vi "Element Edit.vi"(10 "Data":T1, 11 "Project":string) -> (2 "Data Out":T1, 3 "OK?":bool)   [LabVIEW 2020]
uses:
  Global/Data Global/SDQ Data Type.ctl
panel:
  in  "Cancle":bool
  in  "OK":bool
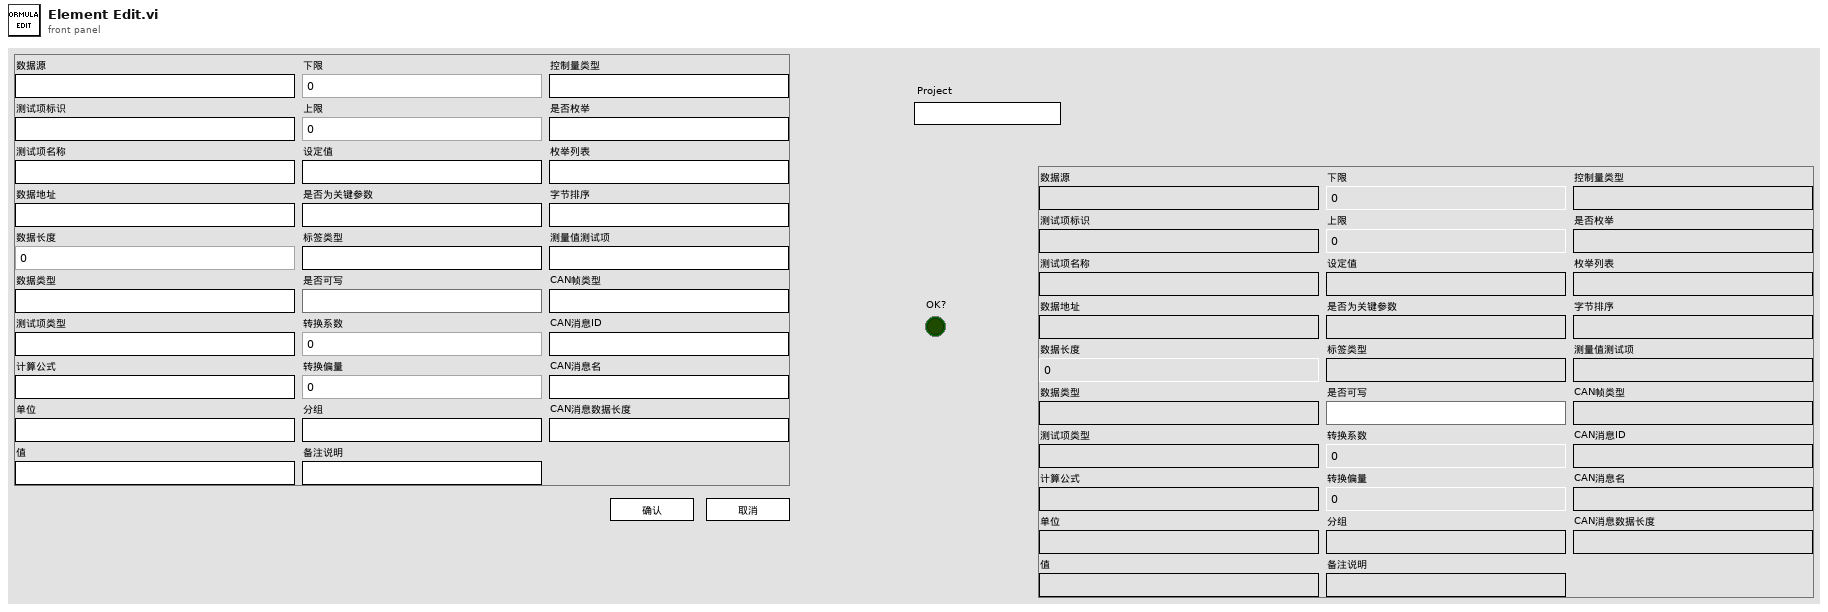
[diagram p1: front panel]
types:
  T1 = typedef "SDQ Data Type.ctl" = cluster{"CAN Length":string, "CAN Name":string, "CAN ID":string, "CAN Type":string, "Test Item":string, "Byte Order":string, "Instruction":string, "Control Type":string, "Group":string, "Offset":dbl, "Coefficient":dbl, "Write Enable":bool, "Lable Type":string, "Key?":string, "Set Value":string, "Upper":dbl, "Lower":dbl, "Unit":string, "Formula":string, "Test Item Type":string, "Length":i32, "Address":string, "Name":string, "Identifier":string, "Data Type":string, "Enumerate?":string, "Enumerate List":string, "Data":string, "Source":string}
  T2 = typedef "eventvkey.ctl" = enum16{"ASCII", "Enter", "Return", "Shift", "Ctrl", "Alt", "Cmd", "Opt", "Caps", "NumLock", "Clear", "Break", "Up", "Down", "Left", "Right", "Insert", "Delete", "Home", "End", "PageUp", "PageDown", "Escape", "Help", "Pause", "ScrollLock", "F1", "F2", "F3", "F4", "F5", "F6", "F7", "F8", "F9", "F10", "F11", "F12", "F13", "F14", "F15", "F16", "F17", "F18", "F19", "F20", "F21", "F22", "F23", "F24", "Play", "VolumeUp", "VolumeDown", "Mute", "Two Byte Char"}
  T3 = cluster{"Project":string, "Element":T1, "OK?":bool}
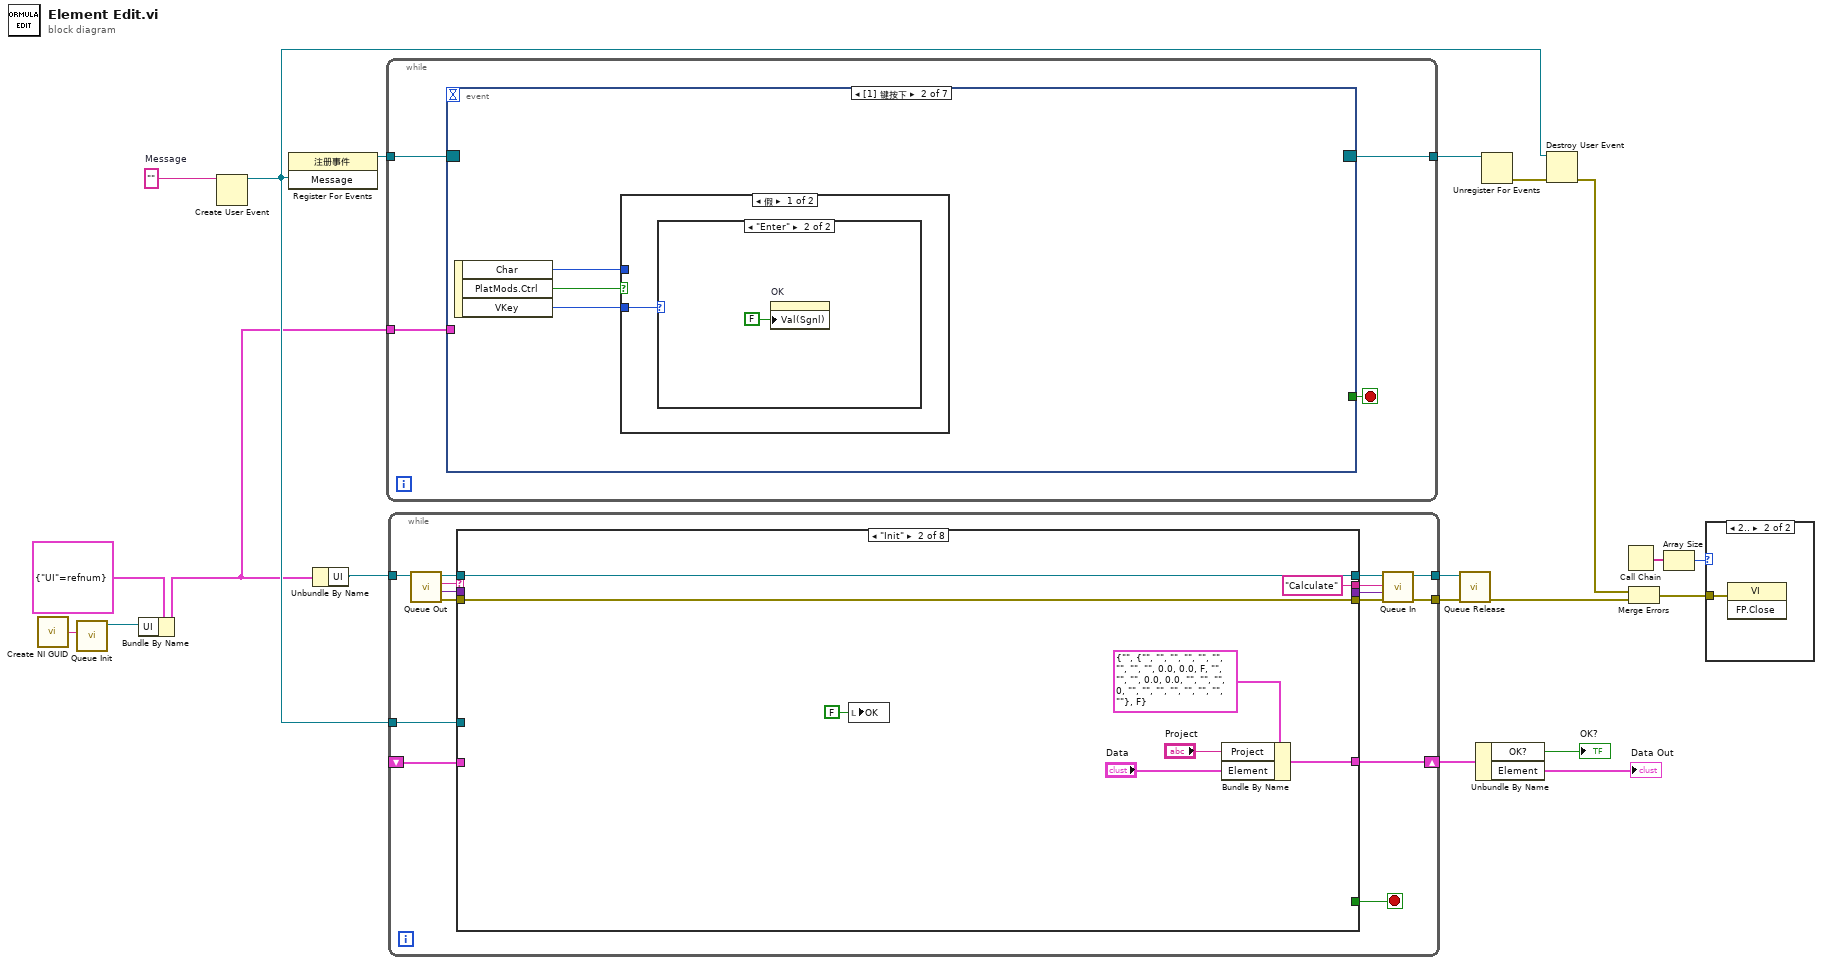
[diagram p0: block diagram]
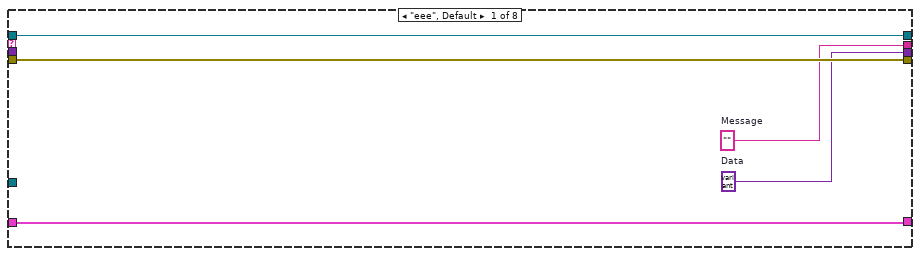
[diagram p3: hidden frame]
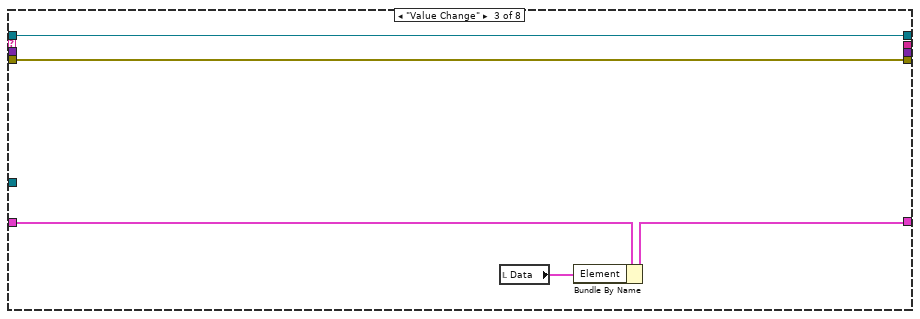
[diagram p4: hidden frame]
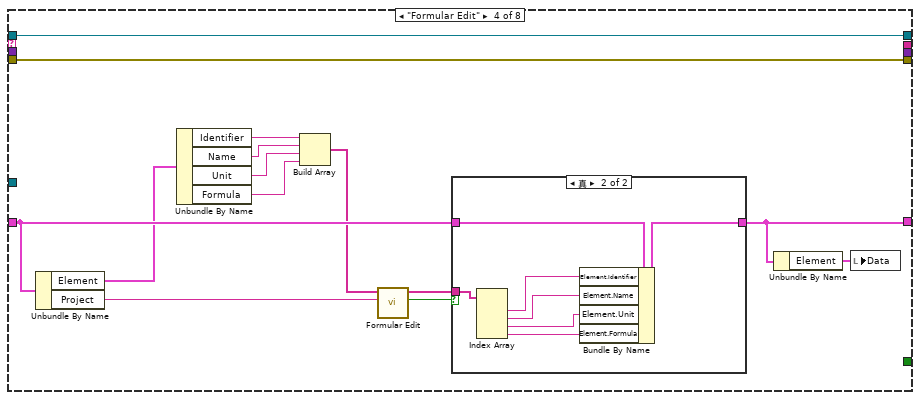
[diagram p5: hidden frame]
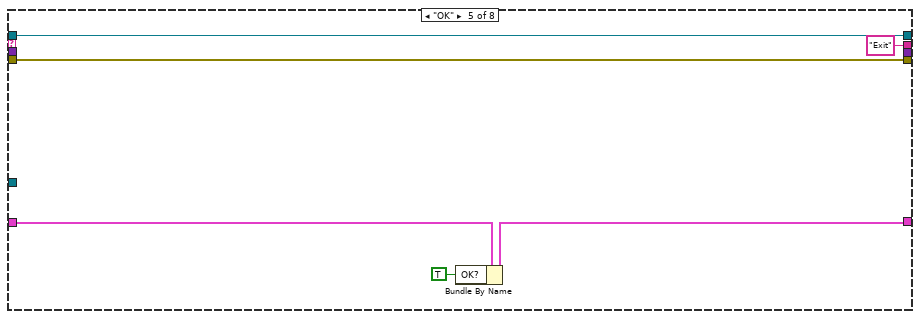
[diagram p7: hidden frame]
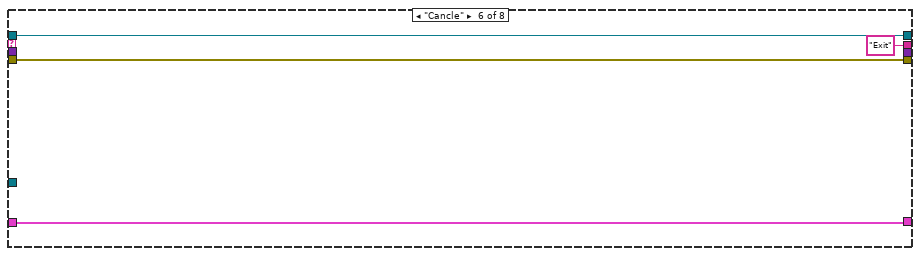
[diagram p8: hidden frame]
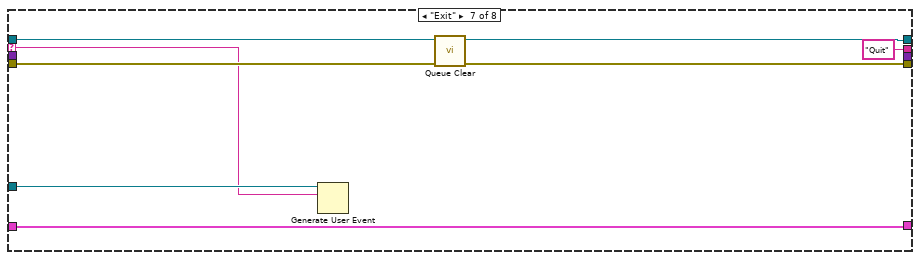
[diagram p9: hidden frame]
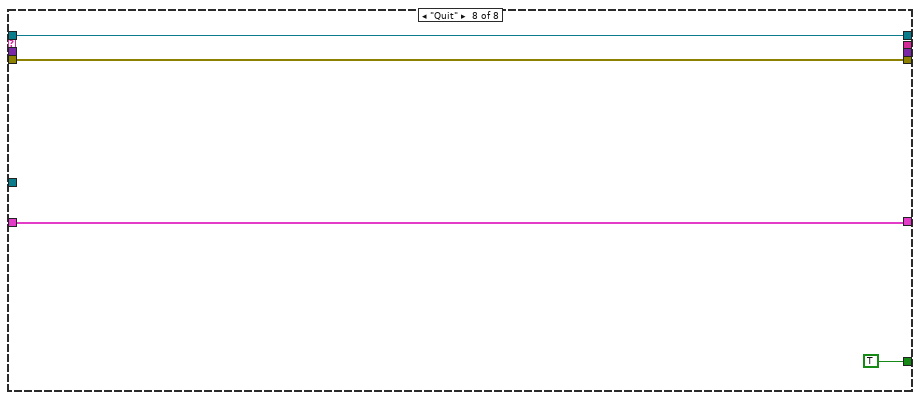
[diagram p10: hidden frame]
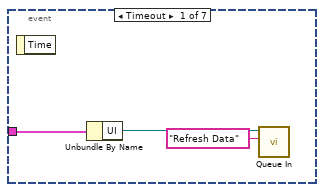
[diagram p11: hidden frame]
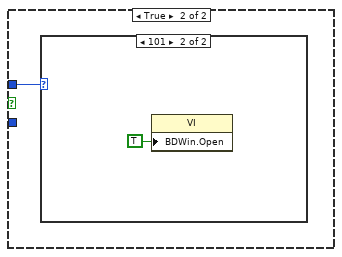
[diagram p13: hidden frame]
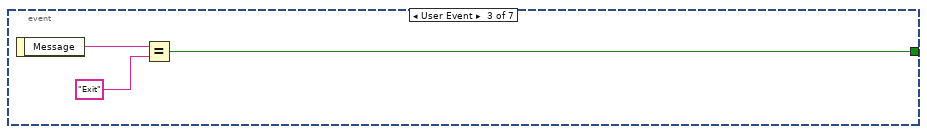
[diagram p15: hidden frame]
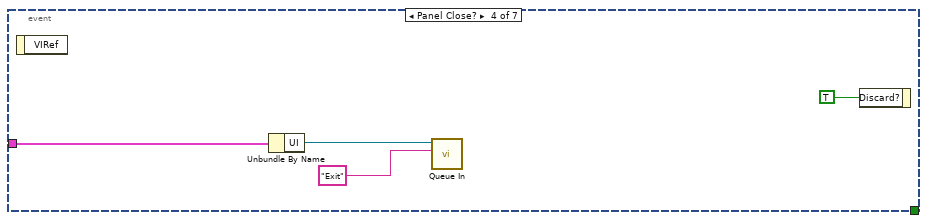
[diagram p16: hidden frame]
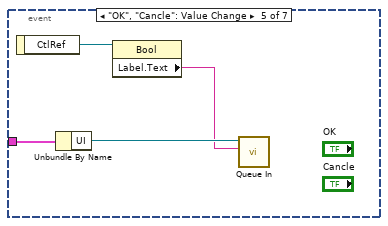
[diagram p17: hidden frame]
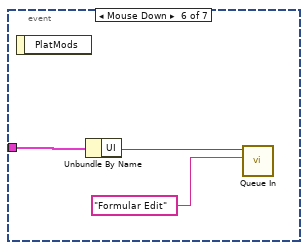
[diagram p18: hidden frame]
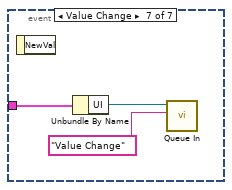
[diagram p19: hidden frame]
diagram:
  w8 = ""  # Message
  n1 = call <vilib>:"Create NI GUID.vi"() -> ("NI GUID"=w6:string)
  n2 = call "Queue Init.vi"("Queue Name"=w6) -> ("Queue Out"=w4:refnum<queue>)  [unwired: 8 in, 2 out]
  n3 = Bundle By Name(cluster=cluster{"UI":refnum<queue>} {"UI"=refnum} ("Queue Ref Out"), "UI"=w4) -> (w5:cluster{"UI":refnum<queue>})
  n4 = Create User Event(user event datatype=w8) -> (user event=w12:refnum<user-event>)  [unwired: 1 in, 1 out]
  n5 = register-events(w12) -> (reference out=w9:refnum<event-registration>)  [unwired: 2 in, 1 out]
  n6 = Unbundle By Name(w5) -> ("UI"=w15:refnum<queue>)
  n7 = while {
    tunnel: w9 -> [w24]
    tunnel: [w22] -> w10
    tunnel: w5 -> [w21]
    stop <- w23 stop-if-true
    n8 = event shown="[1] 键按下" {
      selector: w24 -> [_ _ _ _ _ _ _]
      dyn-events: [_ _ _ _ _ _ _] -> w22
      timeout: _ -> [_ _ _ _ _ _ _]
      tunnel: [_ _ w35 _ _ _ _] -> w23
      tunnel: w21 -> [w27 _ _ w40 w45 w48 w51]
      event Timeout {
        n9 = event-data() -> ()  [unwired: 1 in, 1 out]
        n10 = Unbundle By Name(w27) -> ("UI"=w26:refnum<queue>)
        n11 = call "Queue In.vi"("Message"="Refresh Data", "Queue In"=w26) -> ()  [unwired: 8 in, 2 out]
      }
      event Key Down {
        n12 = event-data() -> ("Char"=w30:i16, "PlatMods.Ctrl"=w29:bool, "VKey"=w28:T2)  [unwired: 1 in]
        n13 = case shown="假" w29 {
          tunnel: w30 -> [_ w33]
          tunnel: w28 -> [w31 _]
          frame False {
            n14 = case shown="\"Enter\"" w31 {
              frame "ASCII", Default {
              }
              frame "Enter" {
                n15 = property on="OK" class="Bool (严格)"("Val(Sgnl)"=FALSE) -> ()  [unwired: 2 in, 2 out]
              }
            }
          }
          frame True {
            n16 = case shown="101" w33 {
              frame 0, Default {
              }
              frame 101 {
                n17 = property class="VI"("BDWin.Open"=TRUE ("程序框图窗口:打开")) -> ()  [unwired: 2 in, 2 out]
              }
            }
          }
        }
      }
      event User Event {
        n18 = event-data() -> ("Message"=w37:string)  [unwired: 1 in]
        n19 = Equal?(x=w37, y="Exit") -> (x = y?=w35:bool)
      }
      event Panel Close? {
        n20 = event-data() -> ()  [unwired: 1 in, 1 out]
        n21 = Unbundle By Name(w40) -> ("UI"=w39:refnum<queue>)
        n22 = call "Queue In.vi"("Message"="Exit", "Queue In"=w39) -> ()  [unwired: 8 in, 2 out]
        n23 = event-data("Discard?"=TRUE ("放弃？")) -> ()  [unwired: 1 in, 1 out]
      }
      event "OK", "Cancle": Value Change {
        n24 = event-data() -> ("CtlRef"=w43:refnum<vi>)  [unwired: 1 in]
        n25 = Unbundle By Name(w45) -> ("UI"=w44:refnum<queue>)
        n26 = property class="Bool"(reference=w43) -> ("Label.Text"=w42:string)  [unwired: 1 in, 2 out]
        n27 = call "Queue In.vi"("Message"=w42, "Queue In"=w44) -> ()  [unwired: 8 in, 2 out]
      }
      event Mouse Down {
        n28 = event-data() -> ()  [unwired: 1 in, 1 out]
        n29 = Unbundle By Name(w48) -> ("UI"=w47:refnum<queue>)
        n30 = call "Queue In.vi"("Message"="Formular Edit", "Queue In"=w47) -> ()  [unwired: 8 in, 2 out]
      }
      event Value Change {
        n31 = event-data() -> ()  [unwired: 1 in, 1 out]
        n32 = Unbundle By Name(w51) -> ("UI"=w50:refnum<queue>)
        n33 = call "Queue In.vi"("Message"="Value Change", "Queue In"=w50) -> ()  [unwired: 8 in, 2 out]
      }
    }
  }
  n34 = while {
    tunnel: w15 -> [w61]
    tunnel: [w58] -> w13
    tunnel: [w57] -> w14
    tunnel: w12 -> [w65]
    shift-right: [w53] -> w3
    shift-left: _ -> [w52]
    stop <- w66 stop-if-true
    n35 = call "Queue Out.vi"("Queue In"=w61) -> ("error out"=w64:errorcluster, "Data"=w62:variant, "Message"=w63:string, "Queue Out"=w60:refnum<queue>)  [unwired: 6 in, 1 out]
    n36 = case shown="\"Init\"" w63 {
      selector: w63 -> [_ _ _ _ _ _ w118 _]
      tunnel: w60 -> [w71 w79 w84 w98 w112 w116 w122 w127]
      tunnel: w64 -> [w70 w78 w83 w97 w111 w115 w120 w128]
      tunnel: [w71 w79 w84 w98 w112 w116 w121 w127] -> w59
      tunnel: [w70 w78 w83 w97 w111 w115 w119 w128] -> w56
      tunnel: [w69 "Calculate" ("Message") _ _ "Exit" ("Message") "Exit" ("Message") "Quit" _] -> w55
      tunnel: [_ _ _ _ _ _ _ TRUE] -> w66
      tunnel: w65 -> [_ _ _ _ _ _ w124 _]
      tunnel: [w68 _ _ _ _ _ _ _] -> w54
      tunnel: w62 -> [_ _ _ _ _ _ _ _]
      tunnel: [w67 w75 w81 w86 w108 w113 w117 w125] -> w53
      tunnel: w52 -> [w67 _ w82 w96 w109 w113 w117 w125]
      frame "eee", Default {
        w68 = variant  # Data
        w69 = ""  # Message
      }
      frame "Init" {
        n37 = local write "OK"(FALSE ("OK")) -> ()
        n38 = Bundle By Name(cluster=T3 {"Project"="", "Element"={"CAN Length"="", "CAN Name"="", "CAN ID"="", "CAN Type"="", "Test Item"="", "Byte Order"="", "Instruction"="", "Control Type"="", "Group"="", "Offset"=0.0, "Coefficient"=0.0, "Write Enable"=FALSE, "Lable Type"="", "Key?"="", "Set Value"="", "Upper"=0.0, "Lower"=0.0, "Unit"="", "Formula"="", "Test Item Type"="", "Length"=0, "Address"="", "Name"="", "Identifier"="", "Data Type"="", "Enumerate?"="", "Enumerate List"="", "Data"="", "Source"=""}, "OK?"=FALSE}, "Project"="Project", "Element"="Data") -> (w75:T3)
      }
      frame "Value Change" {
        n39 = local read "Data"() -> (w80:T1)
        n40 = Bundle By Name(cluster=w82, "Element"=w80) -> (w81:T3)
      }
      frame "Formular Edit" {
        n41 = Unbundle By Name(w96) -> ("Element"=w94:T1, "Project"=w95:string)
        n42 = Unbundle By Name(w94) -> ("Identifier"=w93:string, "Name"=w92:string, "Unit"=w91:string, "Formula"=w90:string)
        n43 = Build Array(w93, w92, w91, w90) -> (w89:string[])
        n44 = call "Formular Edit.vi"("Project"=w95, "Identifier In"=w89) -> ("OK?"=w87:bool, "Identifier In"=w88:string[])  [unwired: 8 in]
        n45 = case shown="真" w87 {
          tunnel: w96 -> [w99 w106]
          tunnel: [w99 w105] -> w86
          tunnel: w88 -> [_ w104]
          frame False {
          }
          frame True {
            n46 = Index Array(array=w104) -> (element #1=w103:string, element #2=w102:string, element #3=w100:string, element #4=w101:string)  [unwired: 4 in]
            n47 = Bundle By Name(cluster=w106, "Element.Identifier"=w103, "Element.Name"=w102, "Element.Unit"=w100, "Element.Formula"=w101) -> (w105:T3)
          }
        }
        n48 = Unbundle By Name(w86) -> ("Element"=w85:T1)
        n49 = local write "Data"(w85) -> ()
      }
      frame "OK" {
        n50 = Bundle By Name(cluster=w109, "OK?"=TRUE) -> (w108:T3)
      }
      frame "Cancle" {
      }
      frame "Exit" {
        n51 = Generate User Event(user event=w124, event data cluster=w118) -> ()  [unwired: 2 in, 2 out]
        n52 = call "Queue Clear.vi"("error in (no error)"=w120, "Queue In"=w122) -> ("error out"=w119:errorcluster, "Queue Out"=w121:refnum<queue>)  [unwired: 8 in]
      }
      frame "Quit" {
      }
    }
    n53 = call "Queue In.vi"("error in (no error)"=w56, "Data"=w54, "Message"=w55, "Queue In"=w59) -> ("error out"=w57:errorcluster, "Queue Out"=w58:refnum<queue>)  [unwired: 6 in]
  }
  n54 = call "Queue Release.vi"("error in (no error)"=w14, "Queue In"=w13) -> ("error out"=w17:errorcluster)  [unwired: 9 in]
  n55 = Unbundle By Name(w3) -> ("OK?"=→"OK?":bool, "Element"=→"Data Out":T1)
  n56 = Unregister For Events(event registration refnum=w10) -> (error out=w11:errorcluster)  [unwired: 1 in]
  n57 = Destroy User Event(user event=w12, error in=w11) -> (error out=w16:errorcluster)
  n58 = Call Chain() -> (call chain=w19:string[])
  n59 = Merge Errors(w16, w17) -> (w18:errorcluster)
  n60 = Array Size(array=w19) -> (size(s)=w20:i32)
  n61 = case shown="2.." w20 {
    tunnel: w18 -> [_ w129]
    frame 0, Default {
    }
    frame 2.. {
      n62 = invoke class="VI" method="FP.Close"(error in=w129) -> ()  [unwired: 2 in, 3 out]
    }
  }
